vi "Convolution with PreSets.vi"(6 "Filter":T1=enum."Seifert 5x5", 8 "error in (no error)":errorcluster, 10 "Image Dst":T2, 11 "Image Src":T2) -> (0 "error out":errorcluster, 1 "Kernel":sgl[][](array[numeric]), 3 "Image Dst Out":T2)   [LabVIEW 2023]
uses:
  <vilib>/vision/Image Controls.llb/IMAQ Image.ctl
  Conv Flt Presets.ctl
  <vilib>/vision/NI_Vision_Development_Module.lvlib
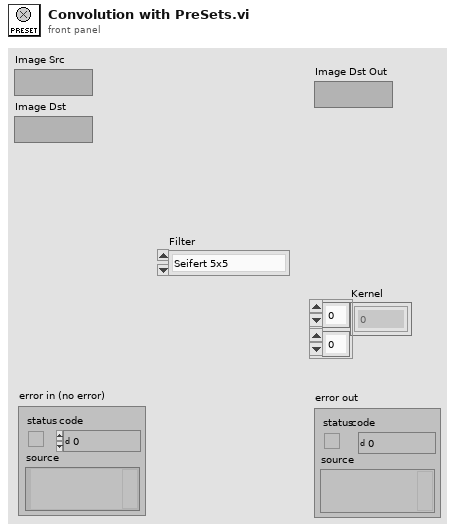
[diagram p1: front panel]
types:
  T1 = typedef "Conv Flt Presets.ctl" = enum16{"None", "Seifert 5x5", "Seifert 7x7", "High Pass 5x5 ", "High Pass 7x7", "Highlight Details 3x3", "Highlight Details 5x5", "Highlight Detail 7x7"}
  T2 = typedef "IMAQ Image.ctl" = refnum<image>
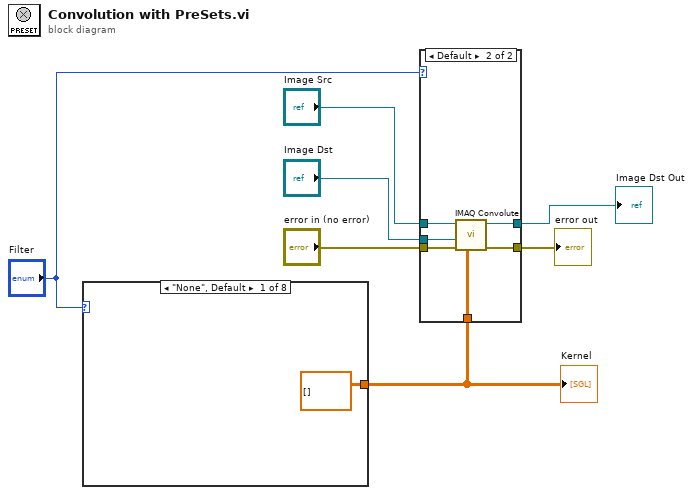
[diagram p0: block diagram]
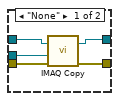
[diagram p2: hidden frame]
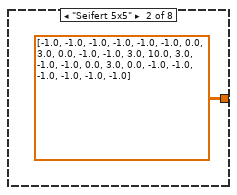
[diagram p3: hidden frame]
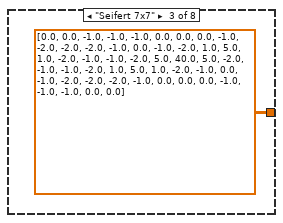
[diagram p4: hidden frame]
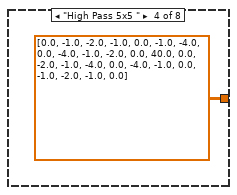
[diagram p5: hidden frame]
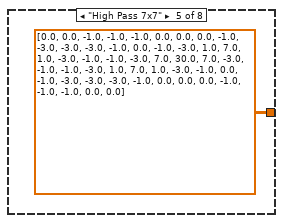
[diagram p6: hidden frame]
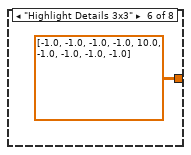
[diagram p7: hidden frame]
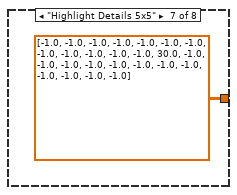
[diagram p8: hidden frame]
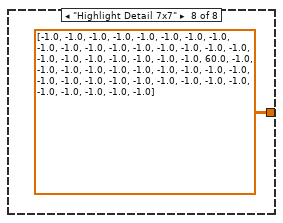
[diagram p9: hidden frame]
diagram:
  n1 = case shown="\"None\", Default" "Filter" {
    tunnel: [sgl[][] [] ("Kernel") sgl[][] [[-1.0, -1.0, -1.0, -1.0, -1.0], [-1.0, 0.0, 3.0, 0.0, -1.0], [-1.0, 3.0, 10.0, 3.0, -1.0], [-1.0, 0.0, 3.0, 0.0, -1.0], [-1.0, -1.0, -1.0, -1.0, -1.0]] ("Kernel") sgl[][] [[0.0, 0.0, -1.0, -1.0, -1.0, 0.0, 0.0], [0.0, -1.0, -2.0, -2.0, -2.0, -1.0, 0.0], [-1.0, -2.0, 1.0, 5.0, 1.0, -2.0, -1.0], [-1.0, -2.0, 5.0, 40.0, 5.0, -2.0, -1.0], [-1.0, -2.0, 1.0, 5.0, 1.0, -2.0, -1.0], [0.0, -1.0, -2.0, -2.0, -2.0, -1.0, 0.0], [0.0, 0.0, -1.0, -1.0, -1.0, 0.0, 0.0]] ("Kernel") sgl[][] [[0.0, -1.0, -2.0, -1.0, 0.0], [-1.0, -4.0, 0.0, -4.0, -1.0], [-2.0, 0.0, 40.0, 0.0, -2.0], [-1.0, -4.0, 0.0, -4.0, -1.0], [0.0, -1.0, -2.0, -1.0, 0.0]] ("Kernel") sgl[][] [[0.0, 0.0, -1.0, -1.0, -1.0, 0.0, 0.0], [0.0, -1.0, -3.0, -3.0, -3.0, -1.0, 0.0], [-1.0, -3.0, 1.0, 7.0, 1.0, -3.0, -1.0], [-1.0, -3.0, 7.0, 30.0, 7.0, -3.0, -1.0], [-1.0, -3.0, 1.0, 7.0, 1.0, -3.0, -1.0], [0.0, -1.0, -3.0, -3.0, -3.0, -1.0, 0.0], [0.0, 0.0, -1.0, -1.0, -1.0, 0.0, 0.0]] ("Kernel") sgl[][] [[-1.0, -1.0, -1.0], [-1.0, 10.0, -1.0], [-1.0, -1.0, -1.0]] ("Kernel") sgl[][] [[-1.0, -1.0, -1.0, -1.0, -1.0], [-1.0, -1.0, -1.0, -1.0, -1.0], [-1.0, -1.0, 30.0, -1.0, -1.0], [-1.0, -1.0, -1.0, -1.0, -1.0], [-1.0, -1.0, -1.0, -1.0, -1.0]] ("Kernel") sgl[][] [[-1.0, -1.0, -1.0, -1.0, -1.0, -1.0, -1.0], [-1.0, -1.0, -1.0, -1.0, -1.0, -1.0, -1.0], [-1.0, -1.0, -1.0, -1.0, -1.0, -1.0, -1.0], [-1.0, -1.0, -1.0, 60.0, -1.0, -1.0, -1.0], [-1.0, -1.0, -1.0, -1.0, -1.0, -1.0, -1.0], [-1.0, -1.0, -1.0, -1.0, -1.0, -1.0, -1.0], [-1.0, -1.0, -1.0, -1.0, -1.0, -1.0, -1.0]] ("Kernel")] -> w4
    frame "None", Default {
    }
    frame "Seifert 5x5" {
    }
    frame "Seifert 7x7" {
    }
    frame "High Pass 5x5 " {
    }
    frame "High Pass 7x7" {
    }
    frame "Highlight Details 3x3" {
    }
    frame "Highlight Details 5x5" {
    }
    frame "Highlight Detail 7x7" {
    }
  }
  "Kernel" <- w4
  n2 = case shown="Default" "Filter" {
    tunnel: "Image Src" -> [w19 w26]
    tunnel: "Image Dst" -> [w18 w25]
    tunnel: [w16 w24] -> w5
    tunnel: w4 -> [_ w23]
    tunnel: "error in (no error)" -> [w17 w22]
    tunnel: [w20 w21] -> w2
    frame "None" {
      n3 = call "IMAQ Copy"("error in (no error)"=w17, "Image Dst"=w18, "Image Src"=w19) -> ("error out"=w20:errorcluster, "Image Dst Out"=w16:T2)  [unwired: 3 in]
    }
    frame Default {
      n4 = call "IMAQ Convolute"("Kernel"=w23, "error in (no error)"=w22, "Image Dst"=w25, "Image Src"=w26) -> ("error out"=w21:errorcluster, "Image Dst Out"=w24:T2)  [unwired: 6 in]
    }
  }
  "Image Dst Out" <- w5
  "error out" <- w2
